vi "Generate_WayPoints_Hopping_DPS_and_CV_with_3segments_V2.vi"(11 "Input Cluster":T2={"X, Y Scan Rate (um/s)"=15.0, "X Start"=15.0, "X End"=15.0, "Y Start"=15.0, "Y End"=15.0, "Z Start"=15.0, "Hopping Distance (um)"=1.0, "V"=15.0, "Z End"=15.0, "Approach Rate Hopping (um/s)"=15.0, "Retrack Rate (um/s)"=15.0, "V2"=15.0, "Approach Rate (um/s)"=15.0, "V3"=15.0, "CV Rate (V/s)"=15.0, "V4"=15.0, "V1"=15.0, "Hold Time1 (ms)"=15.0, "Hold Time2 (ms)"=15.0, "Hold Time3 (ms)"=15.0, "Hold Time4 (ms)"=15.0, "Hold Time5 (ms)"=15.0, "V5"=15.0, "V6"=0.3}) -> (0 "output cluster":T1)   [LabVIEW 2023]
uses:
  TypeDefs/WayPointCluster.ctl
panel:
  in  "WayPointCluster":T1
  out "Y  P":dbl
  out "X  P":dbl
  out "HoppingDistanceX":dbl
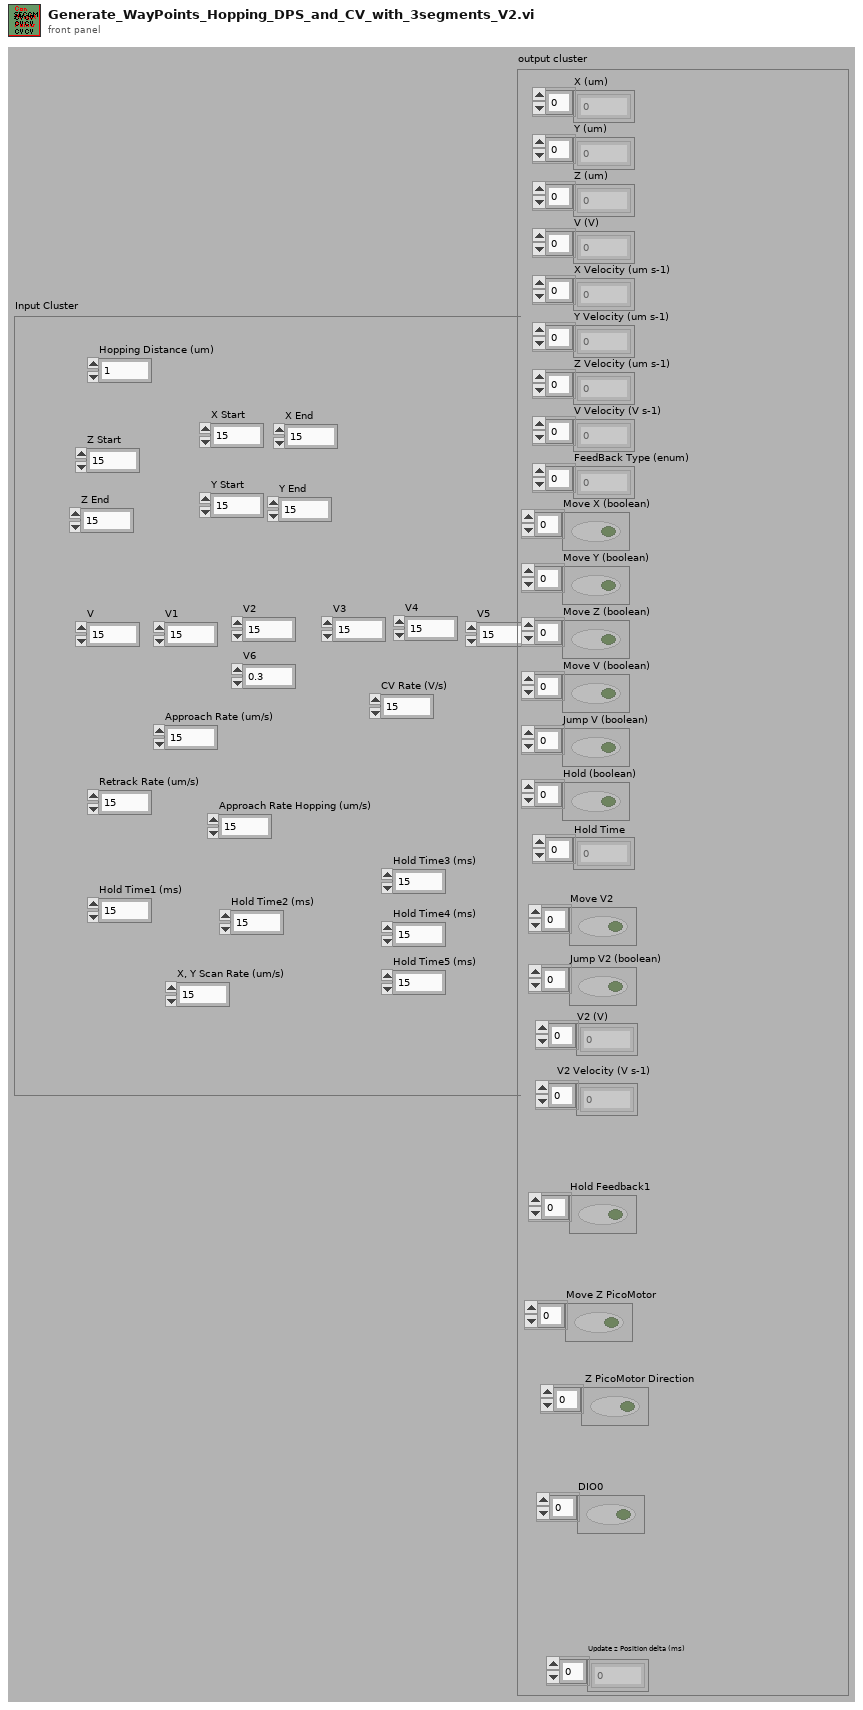
[diagram p1: front panel]
types:
  T1 = typedef "WayPointCluster.ctl" = cluster{"X (um)":dbl[], "Y (um)":dbl[], "Z (um)":dbl[], "V (V)":dbl[], "X Velocity (um s-1)":dbl[], "Y Velocity (um s-1)":dbl[], "Z Velocity (um s-1)":dbl[], "V Velocity (V s-1)":dbl[], "FeedBack Type (enum)":u16[], "Move X (boolean)":bool[], "Move Y (boolean)":bool[], "Move Z (boolean)":bool[], "Move V (boolean)":bool[], "Jump V (boolean)":bool[], "Hold (boolean)":bool[], "Hold Time":u32[], "V2 (V)":dbl[], "Move V2":bool[], "V2 Velocity (V s-1)":dbl[], "Jump V2 (boolean)":bool[], "Update z Position delta (ms)":i16[], "Hold Feedback1":bool[], "Move Z PicoMotor":bool[], " Z PicoMotor Direction":bool[], "DIO0":bool[]}
  T2 = cluster{"X, Y Scan Rate (um/s)":dbl, "X Start":dbl, "X End":dbl, "Y Start":dbl, "Y End":dbl, "Z Start":dbl, "Hopping Distance (um)":dbl, "V":dbl, "Z End":dbl, "Approach Rate Hopping (um/s)":dbl, "Retrack Rate (um/s)":dbl, "V2":dbl, "Approach Rate (um/s)":dbl, "V3":dbl, "CV Rate (V/s)":dbl, "V4":dbl, "V1":dbl, "Hold Time1 (ms)":dbl, "Hold Time2 (ms)":dbl, "Hold Time3 (ms)":dbl, "Hold Time4 (ms)":dbl, "Hold Time5 (ms)":dbl, "V5":dbl, "V6":dbl}
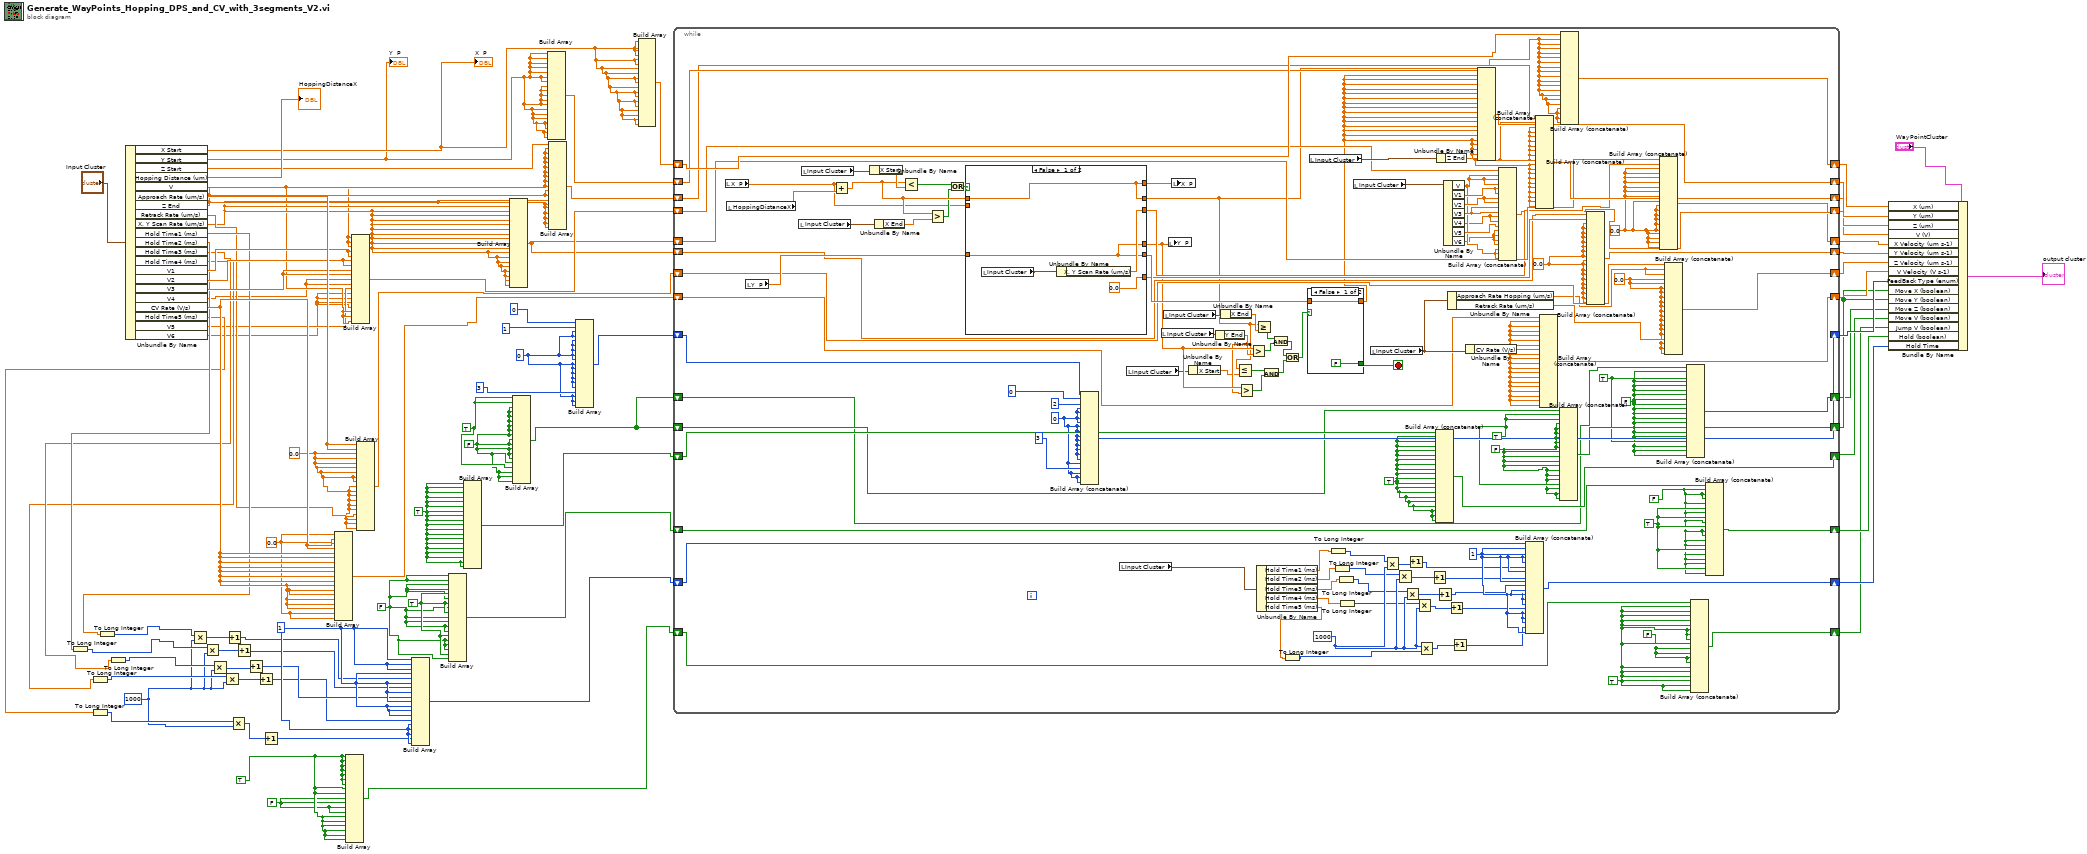
[diagram p0: block diagram]
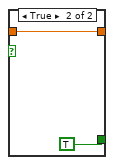
[diagram p2: hidden frame]
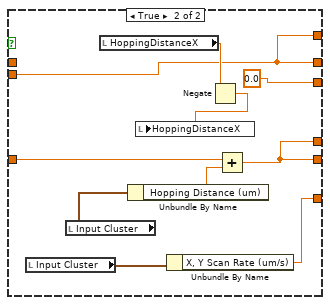
[diagram p3: hidden frame]
diagram:
  w27 = FALSE
  w31 = TRUE
  w22 = 0.0 ("element")
  w34 = u32 1000 ("element")
  w28 = u32 1 ("element")
  w25 = FALSE
  w26 = TRUE
  w20 = FALSE
  w21 = TRUE
  w12 = u16 0 ("element")
  w30 = TRUE
  w29 = 0.0 ("element")
  n1 = Unbundle By Name("Input Cluster") -> ("X Start"=w19:dbl, "Y Start"=w18:dbl, "Z Start"=w58:dbl, "Hopping Distance (um)"=→"HoppingDistanceX":dbl, "V"=w15:dbl, "Approach Rate (um/s)"=w52:dbl, "Z End"=w17:dbl, "Retrack Rate (um/s)"=w23:dbl, "X, Y Scan Rate (um/s)"=w16:dbl, "Hold Time1 (ms)"=w44:dbl, "Hold Time2 (ms)"=w42:dbl, "Hold Time3 (ms)"=w40:dbl, "Hold Time4 (ms)"=w37:dbl, "V1"=w47:dbl, "V2"=w46:dbl, "V3"=w45:dbl, "V4"=w13:dbl, "CV Rate (V/s)"=w48:dbl, "Hold Time5 (ms)"=w36:dbl, "V5"=w14:dbl, "V6"=w11:dbl)
  "X  P" <- w19
  "Y  P" <- w18
  n2 = To Long Integer(number=w42) -> (32bit integer=w41:i32)
  n3 = To Long Integer(number=w37) -> (32bit integer=w38:i32)
  n4 = To Long Integer(number=w36) -> (32bit integer=w35:i32)
  n5 = To Long Integer(number=w44) -> (32bit integer=w43:i32)
  n6 = To Long Integer(number=w40) -> (32bit integer=w39:i32)
  n7 = Multiply(x=w43, y=w34) -> (x*y=w10:u32)
  n8 = Multiply(x=w41, y=w34) -> (x*y=w8:u32)
  n9 = Multiply(x=w39, y=w34) -> (x*y=w6:u32)
  n10 = Multiply(x=w38, y=w34) -> (x*y=w4:u32)
  n11 = Increment(x=w10) -> (x+1=w9:u32)
  n12 = Multiply(x=w35, y=w34) -> (x*y=w2:u32)
  n13 = Increment(x=w8) -> (x+1=w7:u32)
  n14 = Increment(x=w6) -> (x+1=w5:u32)
  n15 = Increment(x=w4) -> (x+1=w3:u32)
  n16 = Increment(x=w2) -> (x+1=w1:u32)
  n17 = Build Array(w29, w29, w48, w48, w48, w48, w48, w48, w48, w48, w48, w48, w48, w48, w48, w48, w48, w29, w29) -> (w50:dbl[])
  n18 = Build Array(w31, w31, w31, w31, w31, w31, w31, w31, w31, w27, w27, w27, w27, w31, w31, w31, w31, w31, w31) -> (w49:bool[])
  n19 = Build Array(w15, w15, w15, w47, w47, w46, w46, w45, w45, w13, w13, w14, w11, w11, w11, w11, w15, w15, w15) -> (w54:dbl[])
  n20 = Build Array(w52, w52, w22, w22, w22, w22, w22, w22, w22, w22, w22, w22, w22, w22, w22, w23, w22, w22, w22) -> (w51:dbl[])
  n21 = Build Array(w28, w28, w28, w28, w9, w28, w7, w28, w5, w28, w28, w28, w28, w3, w28, w28, w28, w1, w28) -> (w55:u32[])
  n22 = Build Array(w25, w25, w25, w25, w26, w25, w26, w25, w26, w25, w25, w25, w25, w26, w25, w25, w25, w26, w25) -> (w56:bool[])
  n23 = Build Array(w30, w30, w30, w30, w30, w30, w30, w30, w30, w30, w30, w30, w30, w30, w30, w30, w30, w30, w30) -> (w57:bool[])
  n24 = Build Array(w16, w16, w16, w16, w16, w16, w16, w16, w16, w16, w16, w16, w16, w16, w16, w16, w16, w16, w16) -> (w53:dbl[])
  n25 = Build Array(w21, w21, w20, w20, w20, w20, w20, w20, w20, w20, w20, w20, w20, w20, w20, w21, w20, w20, w20) -> (w33:bool[])
  n26 = Build Array(w18, w18, w18, w18, w18, w18, w18, w18, w18, w18, w18, w18, w18, w18, w18, w18, w18, w18, w18) -> (w60:dbl[])
  n27 = Build Array(w58, w17, w17, w17, w17, w17, w17, w17, w17, w17, w17, w17, w17, w17, w17, w17, w17, w17, w17) -> (w59:dbl[])
  n28 = Build Array(u16 0 ("element"), u16 1 ("element"), w12, w12, w12, w12, w12, w12, w12, w12, w12, w12, w12, w12, w12, u16 3 ("element"), w12, w12, w12) -> (w73:u16[])
  n29 = Build Array(w19, w19, w19, w19, w19, w19, w19, w19, w19, w19, w19, w19, w19, w19, w19, w19, w19, w19, w19) -> (w61:dbl[])
  n30 = while {
    shift-right: [w174] -> w80
    shift-left: w61 -> [w175]
    shift-right: [w172] -> w79
    shift-left: w60 -> [w173]
    shift-right: [w170] -> w78
    shift-left: w59 -> [w171]
    shift-right: [w163] -> w77
    shift-left: w54 -> [w164]
    shift-right: [w162] -> w70
    shift-left: w53 -> [w169]
    shift-right: [w165] -> w76
    shift-left: w53 -> [w166]
    shift-right: [w160] -> w75
    shift-left: w51 -> [w161]
    shift-right: [w158] -> w74
    shift-left: w50 -> [w159]
    shift-right: [w193] -> w72
    shift-left: w73 -> [w194]
    shift-right: [w157] -> w69
    shift-left: w33 -> [w118]
    shift-right: [w153] -> w68
    shift-left: w56 -> [w154]
    shift-right: [w151] -> w67
    shift-left: w55 -> [w152]
    shift-right: [w148] -> w66
    shift-left: w49 -> [w149]
    shift-right: [w155] -> w64
    shift-left: w57 -> [w156]
    shift-right: [w116] -> w32
    shift-left: w33 -> [w117]
    stop <- w183 stop-if-true
    w104 = FALSE
    w105 = TRUE
    w130 = u32 1000 ("element")
    w115 = TRUE
    w97 = 0.0 ("element")
    w108 = TRUE
    w114 = FALSE
    w113 = u32 1 ("element")
    w112 = TRUE
    w111 = FALSE
    w106 = FALSE
    w107 = TRUE
    w109 = u16 0 ("element")
    w96 = 0.0 ("element")
    w102 = 0.0 ("element")
    n31 = local read "X  P"() -> (w182:dbl)
    n32 = local read "HoppingDistanceX"() -> (w195:dbl)
    n33 = local read "Y  P"() -> (w181:dbl)
    n34 = local read "Input Cluster"() -> (w196:T2)
    n35 = local read "Input Cluster"() -> (w197:T2)
    n36 = Add(x=w182, y=w195) -> (x+y=w187:dbl)
    n37 = Unbundle By Name(w197) -> ("X Start"=w190:dbl)
    n38 = Unbundle By Name(w196) -> ("X End"=w188:dbl)
    n39 = Less?(x=w187, y=w190) -> (x < y?=w189:bool)
    n40 = Greater?(x=w187, y=w188) -> (0:w186:bool)
    n41 = Or(x=w189, y=w186) -> (x .or. y?=w185:bool)
    n42 = case shown="False" w185 {
      tunnel: w187 -> [w202 _]
      tunnel: [w202 w208] -> w99
      tunnel: w182 -> [_ w208]
      tunnel: w181 -> [w203 w209]
      tunnel: [w203 w207] -> w180
      tunnel: [w205 0.0] -> w168
      tunnel: [0.0 w210] -> w167
      tunnel: [w203 w207] -> w136
      tunnel: [w202 w208] -> w179
      frame False {
        n43 = local read "Input Cluster"() -> (w206:T2)
        n44 = Unbundle By Name(w206) -> ("X, Y Scan Rate (um/s)"=w205:dbl)
      }
      frame True {
        n45 = local read "Input Cluster"() -> (w212:T2)
        n46 = local read "Input Cluster"() -> (w214:T2)
        n47 = local read "HoppingDistanceX"() -> (w216:dbl)
        n48 = Unbundle By Name(w214) -> ("Hopping Distance (um)"=w213:dbl)
        n49 = Unbundle By Name(w212) -> ("X, Y Scan Rate (um/s)"=w210:dbl)
        n50 = Negate(x=w216) -> (-x=w215:dbl)
        n51 = local write "HoppingDistanceX"(w215) -> ()
        n52 = Add(x=w209, y=w213) -> (x+y=w207:dbl)
      }
    }
    n53 = Build Array (concatenate)(w194, u16 0 ("element"), u16 2 ("element"), w109, w109, w109, w109, w109, w109, w109, w109, w109, w109, w109, w109, w109, u16 3 ("element"), w109, w109, w109) -> (w193:u16[])
    n54 = local read "Input Cluster"() -> (w150:T2)
    n55 = local read "Input Cluster"() -> (w133:T2)
    n56 = local read "Input Cluster"() -> (w184:T2)
    n57 = local read "Input Cluster"() -> (w143:T2)
    n58 = local write "Y  P"(w136) -> ()
    n59 = local write "X  P"(w179) -> ()
    n60 = Unbundle By Name(w133) -> ("X Start"=w132:dbl)
    n61 = Unbundle By Name(w184) -> ("Y End"=w135:dbl)
    n62 = Unbundle By Name(w143) -> ("X End"=w142:dbl)
    n63 = Less Or Equal?(x=w99, y=w132) -> (x <= y?=w131:bool)
    n64 = Greater?(x=w136, y=w135) -> (0:w134:bool)
    n65 = Greater?(x=w136, y=w135) -> (0:w140:bool)
    n66 = Greater Or Equal?(x=w99, y=w142) -> (x >= y?=w141:bool)
    n67 = Unbundle By Name(w150) -> ("Hold Time1 (ms)"=w129:dbl, "Hold Time2 (ms)"=w126:dbl, "Hold Time3 (ms)"=w125:dbl, "Hold Time4 (ms)"=w123:dbl, "Hold Time5 (ms)"=w121:dbl)
    n68 = And(x=w131, y=w134) -> (x .and. y?=w137:bool)
    n69 = And(x=w141, y=w140) -> (x .and. y?=w139:bool)
    n70 = Or(x=w139, y=w137) -> (x .or. y?=w138:bool)
    n71 = To Long Integer(number=w121) -> (32bit integer=w120:i32)
    n72 = case shown="False" w138 {
      tunnel: w180 -> [w199 w201]
      tunnel: [w199 w201] -> w100
      tunnel: [FALSE TRUE] -> w183
      frame False {
      }
      frame True {
      }
    }
    n73 = local read "Input Cluster"() -> (w192:T2)
    n74 = To Long Integer(number=w129) -> (32bit integer=w128:i32)
    n75 = To Long Integer(number=w126) -> (32bit integer=w127:i32)
    n76 = To Long Integer(number=w125) -> (32bit integer=w124:i32)
    n77 = To Long Integer(number=w123) -> (32bit integer=w122:i32)
    n78 = local read "Input Cluster"() -> (w191:T2)
    n79 = local read "Input Cluster"() -> (w176:T2)
    n80 = Multiply(x=w128, y=w130) -> (x*y=w93:u32)
    n81 = Multiply(x=w127, y=w130) -> (x*y=w91:u32)
    n82 = Multiply(x=w124, y=w130) -> (x*y=w89:u32)
    n83 = Increment(x=w93) -> (x+1=w92:u32)
    n84 = Multiply(x=w122, y=w130) -> (x*y=w87:u32)
    n85 = Multiply(x=w130, y=w120) -> (x*y=w85:u32)
    n86 = Increment(x=w91) -> (x+1=w90:u32)
    n87 = Build Array (concatenate)(w156, w108, w108, w108, w108, w108, w108, w108, w108, w108, w108, w108, w108, w108, w108, w108, w108, w108, w108, w108) -> (w155:bool[])
    n88 = Increment(x=w89) -> (x+1=w88:u32)
    n89 = Unbundle By Name(w192) -> ("Z End"=w98:dbl)
    n90 = Unbundle By Name(w191) -> ("V"=w95:dbl, "V1"=w145:dbl, "V2"=w144:dbl, "V3"=w147:dbl, "V4"=w94:dbl, "V5"=w119:dbl, "V6"=w83:dbl)
    n91 = Unbundle By Name(w176) -> ("Approach Rate Hopping (um/s)"=w146:dbl, "Retrack Rate (um/s)"=w103:dbl)
    n92 = Increment(x=w87) -> (x+1=w86:u32)
    n93 = Increment(x=w85) -> (x+1=w84:u32)
    n94 = Unbundle By Name(w176) -> ("CV Rate (V/s)"=w101:dbl)
    n95 = Build Array (concatenate)(w173, w100, w100, w100, w100, w100, w100, w100, w100, w100, w100, w100, w100, w100, w100, w100, w100, w100, w100, w100) -> (w172:dbl[])
    n96 = Build Array (concatenate)(w164, w95, w95, w95, w145, w145, w144, w144, w147, w147, w94, w94, w119, w83, w83, w83, w83, w95, w95, w95) -> (w163:dbl[])
    n97 = Build Array (concatenate)(w152, w113, w113, w113, w113, w92, w113, w90, w113, w88, w113, w113, w113, w113, w86, w113, w113, w113, w84, w113) -> (w151:u32[])
    n98 = Build Array (concatenate)(w171, w98, w98, w98, w98, w98, w98, w98, w98, w98, w98, w98, w98, w98, w98, w98, w98, w98, w98, w98) -> (w170:dbl[])
    n99 = Build Array (concatenate)(w159, w101, w101, w101, w101, w101, w101, w101, w101, w101, w101, w101, w101, w101, w101, w101, w101, w101, w101, w101) -> (w158:dbl[])
    n100 = Build Array (concatenate)(w118, w107, w107, w106, w106, w106, w106, w106, w106, w106, w106, w106, w106, w106, w106, w106, w107, w106, w106, w106) -> (w157:bool[])
    n101 = Build Array (concatenate)(w175, w99, w99, w99, w99, w99, w99, w99, w99, w99, w99, w99, w99, w99, w99, w99, w99, w99, w99, w99) -> (w174:dbl[])
    n102 = Build Array (concatenate)(w166, w167, w96, w96, w96, w96, w96, w96, w96, w96, w96, w96, w96, w96, w96, w96, w96, w96, w96, w96) -> (w165:dbl[])
    n103 = Build Array (concatenate)(w169, w168, w97, w97, w97, w97, w97, w97, w97, w97, w97, w97, w97, w97, w97, w97, w97, w97, w97, w97) -> (w162:dbl[])
    n104 = Build Array (concatenate)(w161, w146, w146, w102, w102, w102, w102, w102, w102, w102, w102, w102, w102, w102, w102, w102, w103, w102, w102, w102) -> (w160:dbl[])
    n105 = Build Array (concatenate)(w117, w104, w105, w104, w104, w104, w104, w104, w104, w104, w104, w104, w104, w104, w104, w104, w105, w104, w104, w104) -> (w116:bool[])
    n106 = Build Array (concatenate)(w149, w115, w115, w115, w115, w115, w115, w115, w115, w115, w114, w114, w114, w114, w115, w115, w115, w115, w115, w115) -> (w148:bool[])
    n107 = Build Array (concatenate)(w154, w111, w111, w111, w111, w112, w111, w112, w111, w112, w111, w111, w111, w111, w112, w111, w111, w111, w112, w111) -> (w153:bool[])
  }
  n108 = Bundle By Name(cluster="WayPointCluster", "X (um)"=w80, "Y (um)"=w79, "Z (um)"=w78, "V (V)"=w77, "X Velocity (um s-1)"=w70, "Y Velocity (um s-1)"=w76, "Z Velocity (um s-1)"=w75, "V Velocity (V s-1)"=w74, "FeedBack Type (enum)"=w72, "Move X (boolean)"=w69, "Move Y (boolean)"=w69, "Move Z (boolean)"=w32, "Move V (boolean)"=w64, "Jump V (boolean)"=w66, "Hold (boolean)"=w68, "Hold Time"=w67) -> (→"output cluster":T1)
